vi "Tosca-Init AI Graphs.vi"(0 "Digital":refnum<vi>, 1 "VI in":refnum<vi>, 2 "AI":T2, 5 "Analog":refnum<vi>, 7 "Legend":refnum<vi>, 9 "History (s)":dbl, 12 "Pane in":refnum<vi>, 13 "Splitter":refnum<vi>) -> (8 "plot map":T1[](array[typedef]), 15 "first AI":i32)   [LabVIEW 2020]
uses:
  Typedefs/Tosca-AI.ctl
  Typedefs/Tosca-AI Plot Properties.ctl
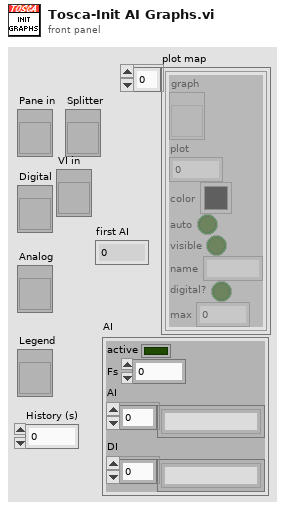
[diagram p1: front panel]
types:
  T1 = typedef "Tosca-AI Plot Properties.ctl" = cluster{"graph":refnum<vi>, "plot":i32, "color":u32, "auto":bool, "visible":bool, "name":string, "digital?":bool, "max":dbl}
  T2 = typedef "Tosca-AI.ctl" = cluster{"active":bool, "Fs":dbl, "AI":string[], "DI":string[]}
  T3 = typedef "LVPointTypeDef.ctl" = cluster{"Horizontal":i16, "Vertical":i16}
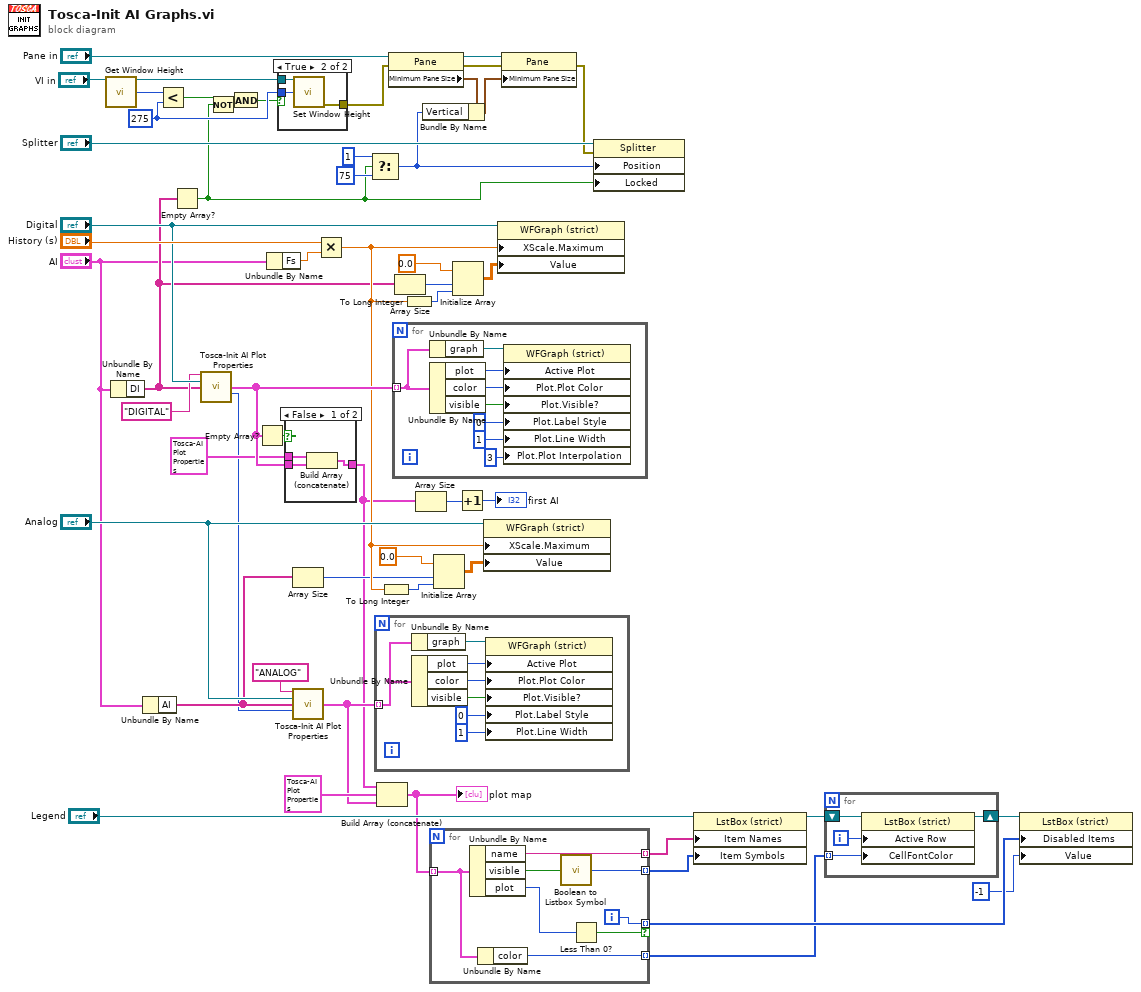
[diagram p0: block diagram]
diagram:
  w6 = 275
  n1 = call "Get Window Height.vi"("VI in"="VI in") -> ("VI out"=w8:refnum<vi>, "Height"=w9:i16)  [unwired: 12 in, 1 out]
  n2 = Unbundle By Name("AI") -> ("DI"=w27:string[])
  n3 = Unbundle By Name("AI") -> ("AI"=w25:string[])
  n4 = Less?(x=w9, y=w6) -> (x < y?=w5:bool)
  n5 = Empty Array?(array=w27) -> (empty?=w4:bool)
  n6 = call "Tosca-Init AI Plot Properties.vi"("which kind"="DIGITAL", "graph"="Digital", "names"=w27) -> ("map"=w35:T1[], "next color"=w1:i32)  [unwired: 10 in, 1 out]
  n7 = Not(x=w4) -> (.not. x?=w3:bool)
  n8 = And(x=w5, y=w3) -> (x .and. y?=w2:bool)
  n9 = Empty Array?(array=w35) -> (empty?=w36:bool)
  n10 = Unbundle By Name("AI") -> ("Fs"=w44:dbl)
  n11 = case shown="True" w2 {
    tunnel: w8 -> [_ w58]
    tunnel: [_ w57] -> w7
    tunnel: w6 -> [_ w56]
    frame False {
    }
    frame True {
      n12 = call "Set Window Height.vi"("VI in"=w58, "Height"=w56) -> ("error out"=w57:errorcluster)  [unwired: 12 in, 1 out]
    }
  }
  n13 = case shown="False" w36 {
    tunnel: w35 -> [w61 w62]
    tunnel: [w60 w62] -> w13
    tunnel: T1 {"graph"=refnum, "plot"=-1, "color"=16448250, "auto"=FALSE, "visible"=FALSE, "name"="DIGITAL", "digital?"=FALSE, "max"=0.0} -> [w59 _]
    frame False {
      n14 = Build Array (concatenate)(w59, w61) -> (w60:T1[])
    }
    frame True {
    }
  }
  n15 = Array Size(array=w25) -> (size(s)=w17:i32)
  n16 = call "Tosca-Init AI Plot Properties.vi"("which kind"="ANALOG", "graph"="Analog", "names"=w25, "first color"=w1) -> ("map"=w24:T1[])  [unwired: 9 in, 2 out]
  n17 = Multiply(x="History (s)", y=w44) -> (x*y=w28:dbl)
  n18 = Select(t=1, s=w4, f=75) -> (s? t:f=w46:i32)
  n19 = for {
    tunnel: w24 -> [w66] mode=indexing
    n20 = Unbundle By Name(w66) -> ("graph"=w67:refnum<vi>)
    n21 = Unbundle By Name(w66) -> ("plot"=w65:i32, "color"=w64:u32, "visible"=w63:bool)
    n22 = property class="WFGraph (strict)"(reference=w67, "Active Plot"=w65, "Plot.Plot Color"=w64, "Plot.Visible?"=w63, "Plot.Label Style"=u8 0 ("Plot.Digital Line Style"), "Plot.Line Width"=u8 1) -> ()  [unwired: 1 in, 2 out]
  }
  n23 = Build Array (concatenate)(w13, T1 {"graph"=refnum, "plot"=-1, "color"=16448250, "auto"=FALSE, "visible"=FALSE, "name"="ANALOG", "digital?"=FALSE, "max"=0.0}, w24) -> (w23:T1[])
  "plot map" <- w23
  n24 = To Long Integer(number=w28) -> (32bit integer=w18:i32)
  n25 = property class="Pane"(reference="Pane in", error in=w7) -> (reference out=w51:refnum<vi>, error out=w48:errorcluster, "Minimum Pane Size"=w52:T3)
  n26 = for {
    tunnel: w35 -> [w74] mode=indexing
    n27 = Unbundle By Name(w74) -> ("graph"=w75:refnum<vi>)
    n28 = Unbundle By Name(w74) -> ("plot"=w73:i32, "color"=w72:u32, "visible"=w71:bool)
    n29 = property class="WFGraph (strict)"(reference=w75, "Active Plot"=w73, "Plot.Plot Color"=w72, "Plot.Visible?"=w71, "Plot.Label Style"=u8 0 ("Plot.Digital Line Style"), "Plot.Line Width"=u8 1, "Plot.Plot Interpolation"=u8 3) -> ()  [unwired: 1 in, 2 out]
  }
  n30 = Array Size(array=w27) -> (size(s)=w15:i32)
  n31 = To Long Integer(number=w28) -> (32bit integer=w16:i32)
  n32 = Array Size(array=w13) -> (size(s)=w12:i32)
  n33 = Bundle By Name(cluster=w52, "Vertical"=w46) -> (w50:T3)
  n34 = for {
    tunnel: w23 -> [w81] mode=indexing
    tunnel: [w85] -> w22 mode=indexing
    tunnel: [w84] -> w21 mode=indexing if=w82
    tunnel: [w80] -> w19 mode=indexing
    tunnel: [w78] -> w14 mode=indexing
    i -> [w84]
    n35 = Unbundle By Name(w81) -> ("name"=w85:string, "visible"=w79:bool, "plot"=w83:i32)
    n36 = Unbundle By Name(w81) -> ("color"=w80:u32)
    n37 = call "Boolean to Listbox Symbol.vi"("Boolean"=w79) -> ("Symbol"=w78:i32)  [unwired: 14 in]
    n38 = Less Than 0?(x=w83) -> (x < 0?=w82:bool)
  }
  n39 = Initialize Array(0.0, w17, w18) -> (w29:dbl[][])
  n40 = Initialize Array(0.0, w15, w16) -> (w39:dbl[][])
  n41 = Increment(x=w12) -> (x+1=→"first AI":i32)
  n42 = property class="WFGraph (strict)"(reference="Analog", "XScale.Maximum"=w28, "Value"=w29) -> ()  [unwired: 1 in, 2 out]
  n43 = property class="WFGraph (strict)"(reference="Digital", "XScale.Maximum"=w28, "Value"=w39) -> ()  [unwired: 1 in, 2 out]
  n44 = property class="Pane"(reference=w51, error in=w48, "Minimum Pane Size"=w50) -> (error out=w49:errorcluster)  [unwired: 1 out]
  n45 = property class="Splitter"(reference="Splitter", error in=w49, "Position"=w46, "Locked"=w4) -> ()  [unwired: 2 out]
  n46 = property class="LstBox (strict)"(reference="Legend", "Item Names"=w22, "Item Symbols"=w14) -> (reference out=w43:refnum<vi>)  [unwired: 1 in, 1 out]
  n47 = for {
    shift-right: [w87] -> w40
    shift-left: w43 -> [w88]
    tunnel: w19 -> [w86] mode=indexing
    i -> [w89]
    n48 = property class="LstBox (strict)"(reference=w88, "Active Row"=w89, "CellFontColor"=w86) -> (reference out=w87:refnum<vi>)  [unwired: 1 in, 1 out]
  }
  n49 = property class="LstBox (strict)"(reference=w40, "Disabled Items"=w21, "Value"=-1 ("Active Row:Active Row Number")) -> ()  [unwired: 1 in, 2 out]
